vi "HSVCombIntensityLifetime.vi"(5 "min_intensity":dbl, 6 "Auto Scale?":bool, 7 "max_intensity":dbl, 8 "lifetime_max (s)":dbl=1e-05, 9 "lifetime_min (s)":dbl, 10 "Lifetime image":dbl[][](array[numeric]), 11 "Intensity image":dbl[][](array[numeric])) -> (0 "Min":dbl=0.001848886980185905, 1 "Max":dbl=0.003482028663545093, 2 "Lifetime Color Ramp":i32[][](graph) caption="Vertical Color Ramp", 3 "HSV to RGB Picture":picture)   [LabVIEW 2018]
uses:
  <vilib>/picture/picture.llb/Draw True-Color Pixmap.vi
panel:
  in  "hue_min [red]":dbl
  in  "hue_max [blue]":dbl=0.7
  # "Local variables"
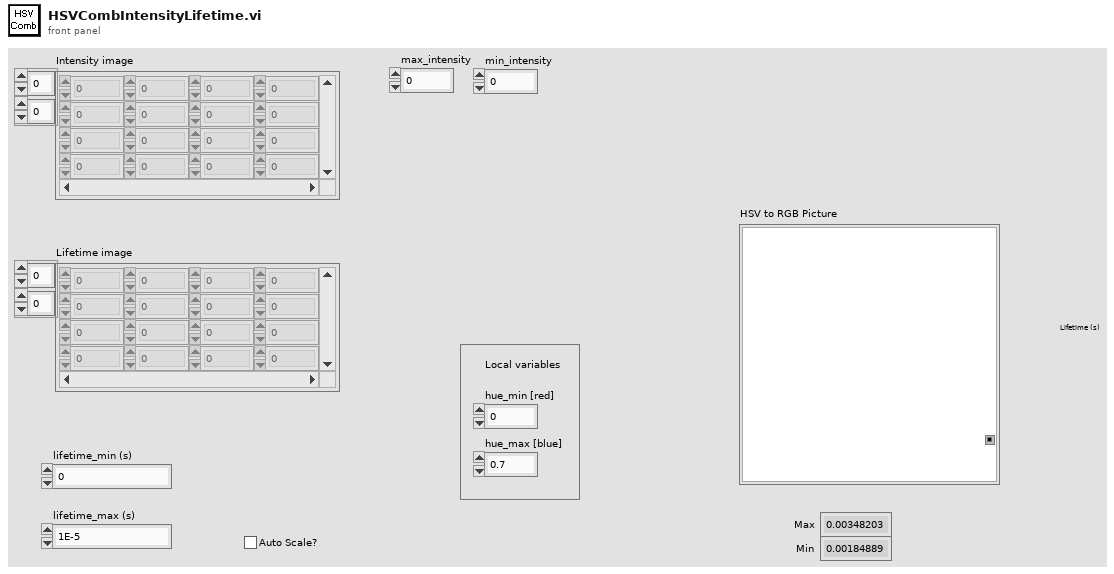
[diagram p1: front panel]
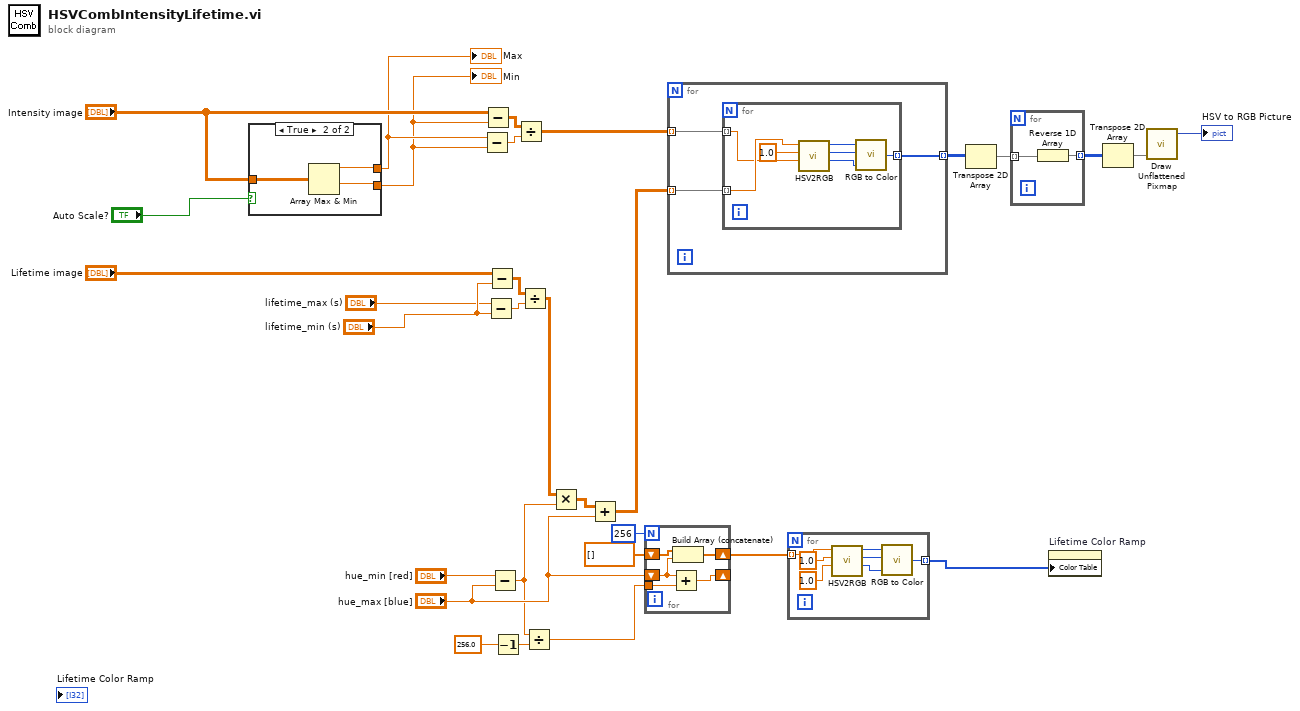
[diagram p0: block diagram]
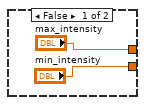
[diagram p2: hidden frame]
diagram:
  n1 = case shown="True" "Auto Scale?" {
    tunnel: "Intensity image" -> [_ w35]
    tunnel: ["max_intensity" w34] -> w3
    tunnel: ["min_intensity" w33] -> w2
    frame False {
    }
    frame True {
      n2 = Array Max & Min(array=w35) -> (max value=w34:dbl, min value=w33:dbl)  [unwired: 2 out]
    }
  }
  "Min" <- w2
  "Max" <- w3
  n3 = Subtract(x=w3, y=w2) -> (x-y=w30:dbl)
  n4 = Subtract(x="Intensity image", y=w2) -> (x-y=w29:dbl[][])
  n5 = Subtract(x="lifetime_max (s)", y="lifetime_min (s)") -> (x-y=w27:dbl)
  n6 = Subtract(x="Lifetime image", y="lifetime_min (s)") -> (x-y=w28:dbl[][])
  n7 = Subtract(x="hue_min [red]", y="hue_max [blue]") -> (x-y=w17:dbl)
  n8 = Decrement(x=256.0) -> (x-1=w25:dbl)
  n9 = Divide(x=w29, y=w30) -> (x/y=w26:dbl[][])
  n10 = Divide(x=w28, y=w27) -> (x/y=w16:dbl[][])
  n11 = Divide(x=w17, y=w25) -> (x/y=w23:dbl)
  n12 = Multiply(x=w16, y=w17) -> (x*y=w15:dbl[][])
  n13 = Add(x=w15, y="hue_max [blue]") -> (x+y=w14:dbl[][])
  n14 = for {
    N: 256 -> [_]
    tunnel: w23 -> [w40]
    shift-right: [w39] -> _
    shift-left: "hue_max [blue]" -> [w36]
    shift-right: [w38] -> w22
    shift-left: dbl[] [] -> [w37]
    n15 = Add(x=w36, y=w40) -> (x+y=w39:dbl)
    n16 = Build Array (concatenate)(w37, w36) -> (w38:dbl[])
  }
  n17 = for {
    tunnel: w26 -> [w43] mode=indexing
    tunnel: [w42] -> w8 mode=indexing
    tunnel: w14 -> [w41] mode=indexing
    n18 = for {
      tunnel: w43 -> [w47] mode=indexing
      tunnel: [w50] -> w42 mode=indexing
      tunnel: w41 -> [w48] mode=indexing
      n19 = call "HSV2RGB.vi"("Value"=w47, "Saturation"=1.0, "Hue [0-1)"=w48) -> ("Blue"=w45:u8, "Green"=w44:u8, "Red"=w46:u8)  [unwired: 6 in]
      n20 = call <vilib>:"RGB to Color.vi"("B"=w45, "G"=w44, "R"=w46) -> ("Color"=w50:u32)
    }
  }
  n21 = for {
    tunnel: [w57] -> w13 mode=indexing
    tunnel: w22 -> [w56] mode=indexing
    n22 = call "HSV2RGB.vi"("Value"=1.0, "Saturation"=1.0, "Hue [0-1)"=w56) -> ("Blue"=w52:u8, "Green"=w53:u8, "Red"=w54:u8)  [unwired: 6 in]
    n23 = call <vilib>:"RGB to Color.vi"("B"=w52, "G"=w53, "R"=w54) -> ("Color"=w57:u32)
  }
  n24 = Transpose 2D Array(2D array=w8) -> (transposed array=w7:u32[][])
  n25 = for {
    tunnel: w7 -> [w59] mode=indexing
    tunnel: [w58] -> w6 mode=indexing
    n26 = Reverse 1D Array(array=w59) -> (reversed array=w58:u32[])
  }
  n27 = property on="Lifetime Color Ramp" class="IntGraph (strict)"("Color Table"=w13) -> ()  [unwired: 2 in, 2 out]
  n28 = Transpose 2D Array(2D array=w6) -> (transposed array=w1:u32[][])
  n29 = call-poly <vilib>:"Draw Unflattened Pixmap.vi"("data (RGB format)"=w1) -> ("new picture"=→"HSV to RGB Picture":picture)  [unwired: 8 in]
